vi "Tömb_összekeverés.vi"(9 "Sorok száma":i32, 10 "Keverendõ tömb(1D)":string[](array[string]), 11 "Sorsolás ism. száma":i32) -> (3 "Összekevert tömb":string[](array[string]))   [LabVIEW 2014]
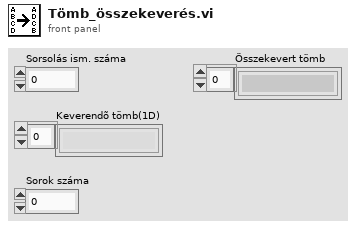
[diagram p1: front panel]
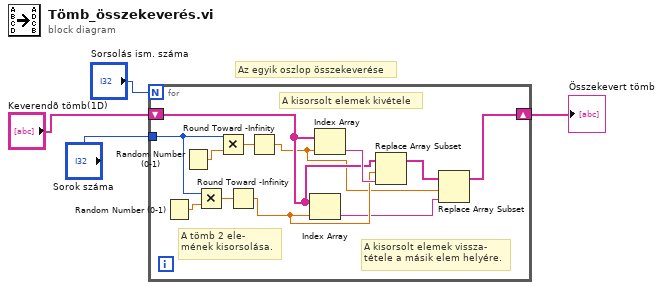
[diagram p0: block diagram]
diagram:
  # "Az egyik oszlop összekeverése"
  n1 = for {
    N: "Sorsolás ism. száma" -> [_]
    tunnel: "Sorok száma" -> [w12]
    shift-right: [w5] -> w3
    shift-left: "Keverendõ tömb(1D)" -> [w10]
    # "A kisorsolt elemek vissza-\ntétele a másik elem helyére."
    # "A tömb 2 ele-\nmének kisorsolása."
    # "A kisorsolt elemek kivétele"
    n2 = Random Number (0-1)() -> (number: 0 to 1=w13:dbl)
    n3 = Random Number (0-1)() -> (number: 0 to 1=w16:dbl)
    n4 = Multiply(x=w12, y=w13) -> (x*y=w15:dbl)
    n5 = Multiply(x=w12, y=w16) -> (x*y=w14:dbl)
    n6 = Round Toward -Infinity(1:w15) -> (0:w9:dbl)
    n7 = Round Toward -Infinity(1:w14) -> (0:w6:dbl)
    n8 = Index Array(array=w10, index=w9) -> (element=w7:string)
    n9 = Index Array(array=w10, index=w6) -> (element=w11:string)
    n10 = Replace Array Subset(array=w10, new element=w11, index=w9) -> (w8:string[])
    n11 = Replace Array Subset(array=w8, new element=w7, index=w6) -> (w5:string[])
  }
  "Összekevert tömb" <- w3
